vi "ELVIS III v1.0 Build MUX Configuration UART.vi"(11 "VISA resource name in":refnum<visa-resource-name>) -> (2 "Channel Reservation List":T1)   [LabVIEW 2021]
uses:
  <vilib>/myRIO/Common/Instrument Driver Framework/ELVIS III v1.0/Resource Manager/typedefs/ELVIS III v1.0 Channel Reservation List.ctl
  <vilib>/myRIO/Common/Instrument Driver Framework/ELVIS III v1.0/Resource Manager/typedefs/ELVIS III v1.0 Channel Reservation Info.ctl
  <vilib>/myRIO/Common/Instrument Driver Framework/ELVIS III v1.0/Resource Manager/typedefs/ELVIS III v1.0 Connector List.ctl
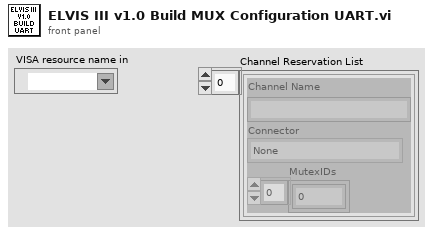
[diagram p1: front panel]
types:
  T1 = typedef "ELVIS III v1.0 Channel Reservation List.ctl" = T2[]
  T2 = typedef "ELVIS III v1.0 Channel Reservation Info.ctl" = cluster{"Channel Name":string, "Connector":T3, "MutexIDs":u32[]}
  T3 = typedef "ELVIS III v1.0 Connector List.ctl" = enum32{"None", "ConnectorA", "ConnectorB"}
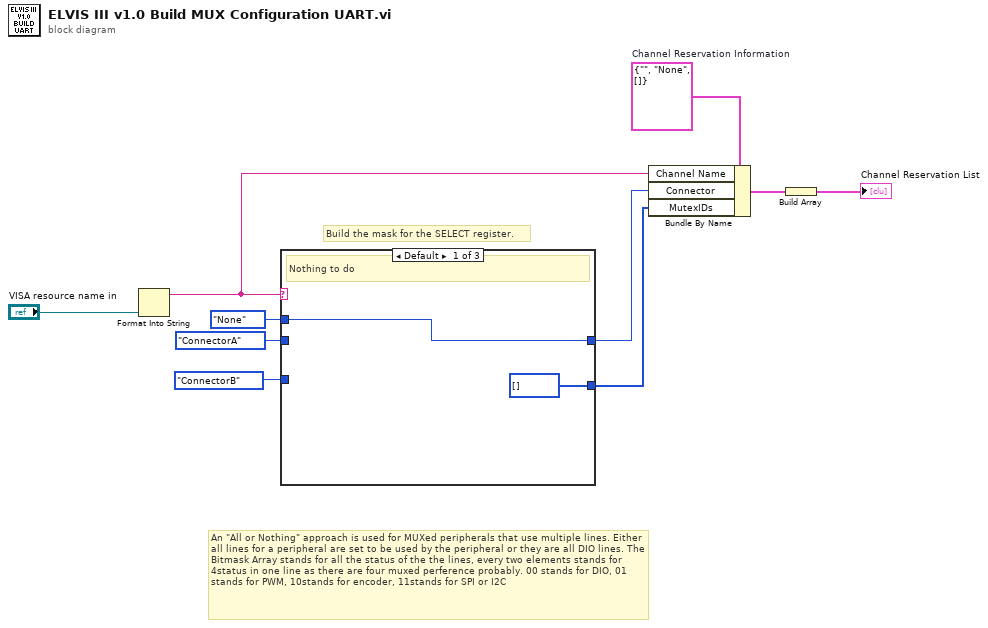
[diagram p0: block diagram]
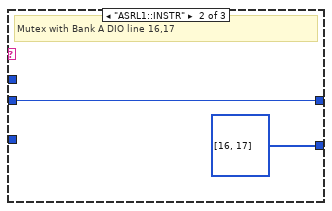
[diagram p2: hidden frame]
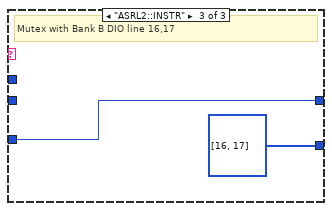
[diagram p3: hidden frame]
diagram:
  w6 = T2 {"Channel Name"="", "Connector"=enum."None", "MutexIDs"=[]}  # Channel Reservation Information
  # "An \"All or Nothing\" approach is used for MUXed peripherals that use multiple lines. Either all lines for a peripheral are set to be used by the peripheral or they are all DIO lines. The Bitmask Array stands for all the status of the the lines, every two elements stands for 4status in one line as there are four muxed perference probably. 00 stands for DIO, 01 stands for PWM, 10stands for encoder, 11stands for SPI or I2C"
  # "Build the mask for the SELECT register."
  n1 = Format Into String("VISA resource name in") -> (resulting string=w1:string)  [unwired: 3 in, 1 out]
  n2 = case shown="Default" w1 {
    tunnel: ELVIS_III_v1.0_Connector_List."None" ("Connector List") -> [w12 _ _]
    tunnel: ELVIS_III_v1.0_Connector_List."ConnectorA" ("Connector List") -> [_ w14 _]
    tunnel: [w12 w14 w16] -> w7
    tunnel: ELVIS_III_v1.0_Connector_List."ConnectorB" ("Connector List") -> [_ _ w16]
    tunnel: [u32[] [] u32[] [16, 17] u32[] [16, 17]] -> w3
    frame Default {
      # "Nothing to do"
    }
    frame "ASRL1::INSTR" {
      # "Mutex with Bank A DIO line 16,17"
    }
    frame "ASRL2::INSTR" {
      # "Mutex with Bank B DIO line 16,17"
    }
  }
  n3 = Bundle By Name(cluster=w6, "Channel Name"=w1, "Connector"=w7, "MutexIDs"=w3) -> (w8:T2)
  n4 = Build Array(w8) -> (→"Channel Reservation List":T2[])
